vi "Client Example.vi"() -> ()   [LabVIEW 2016]
uses:
  <vilib>/NI/STM/SubVIs/MetaDataElement.ctl
  <vilib>/NI/STM/TCP/Read Meta Data (TCP Ref).vi
  <vilib>/NI/STM/TCP/Get Connection Reference (TCP).vi
  <vilib>/NI/STM/TCP/Read Meta Data (TCP Clst).vi
  <vilib>/NI/STM/TCP/Write Message (TCP).vi
  <vilib>/NI/STM/TCP/Read Message (TCP).vi
  <vilib>/NI/STM/NI STM.lvlib
panel:
  out "meta data":T1[](array[typedef])
  in  "Target IP Address":string="localhost"
  in  "Send":bool
  in  "Command":string
  in  "stop":bool
  out "command data string":string
  out "command name":string
  out "error  out":errorcluster
  # "ACTION"
  # "DEBUG"
  # "Set Server IP address (localhost default). \nRun VI. \nSend commands using SEND button, \nreceive ACKs in Debug indicators"
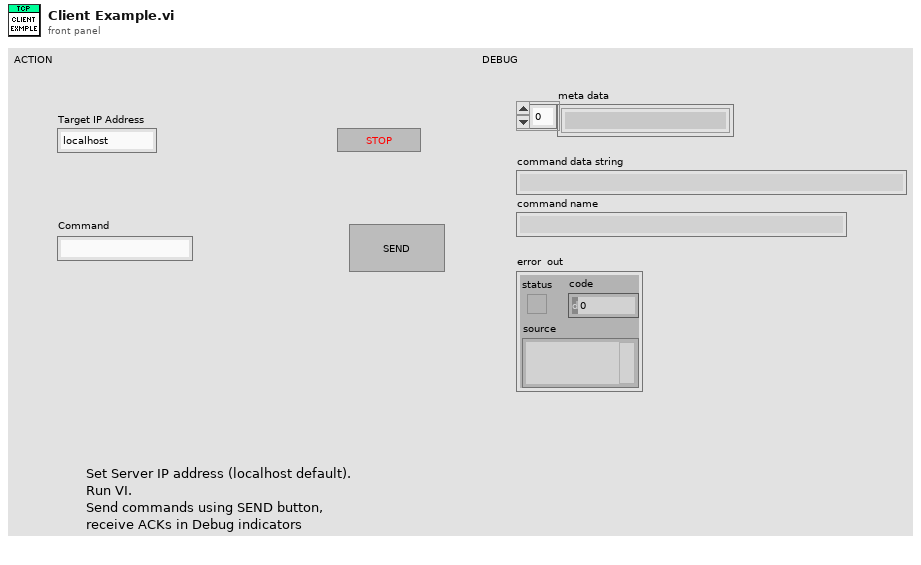
[diagram p1: front panel]
types:
  T1 = typedef "NI STM.lvlib/MetaDataElement.ctl" = string
  T2 = typedef "NI STM.lvlib/TCP Connection Info.ctl" = cluster{"connection ID":refnum<k5>, "meta data":T1[]}
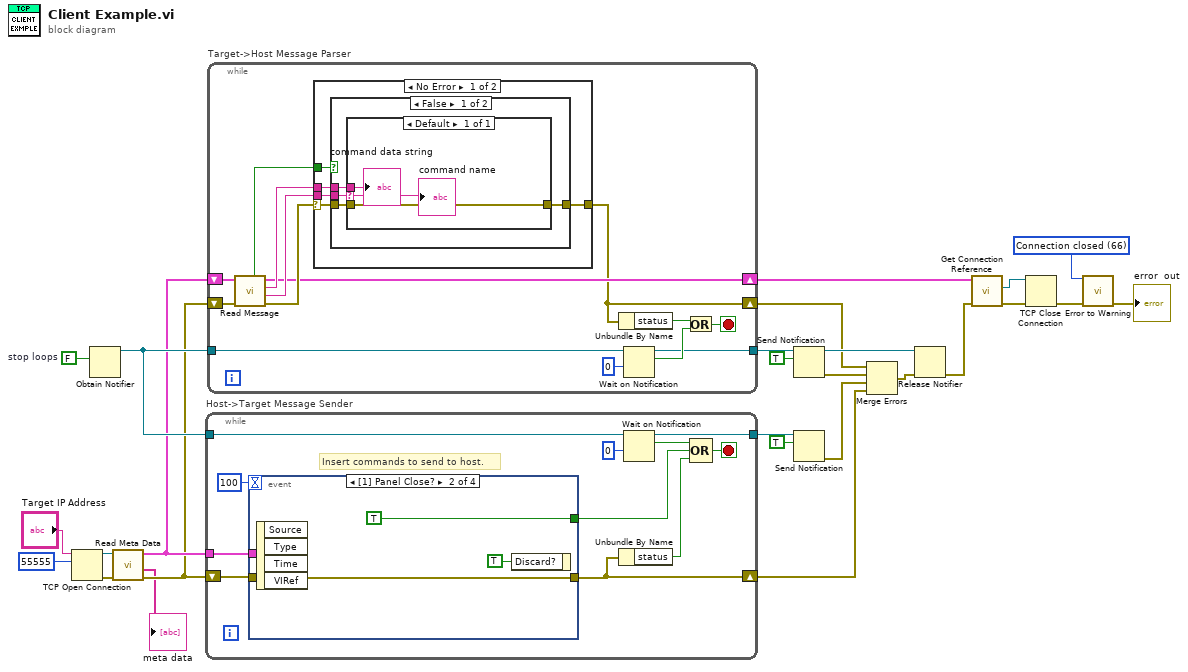
[diagram p0: block diagram]
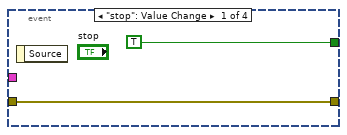
[diagram p2: hidden frame]
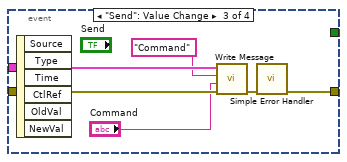
[diagram p3: hidden frame]
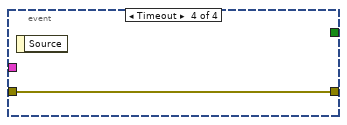
[diagram p4: hidden frame]
diagram:
  w12 = FALSE  # stop loops
  w24 = 66 items=["No Error", "Argument Error", "Memory Full", "Out of Zone", "End of File", "File Already Open", "Generic File IO Error", "File Not Found", "File Permission Error", "Disk Full", "Duplicate Path", "Too Many Files Open", "Not Enabled", "Resource File Not Found", "Cannot Add Resource", "Resource Not Found", "Image Not Found", "Image Memory Error", "Pen Does Not Exist", "Config Bad Type", "Config Token Not Found", "Config Parse Error", "Config Memory Error", "Bad External Code Format", "Bad External Code Offset", "External Code Not Present", "Null Window", "Destroy Window Mixup", "Null Menu", "Print Aborted", "Bad Print Record", "Print Driver Error", "Windows Error During Print", "Memory Error During Print", "Print Dialog Error", "Generic Print Error", "Invalid Device Refnum", "Device Not Found", "Device Parameter Error", "Device Unit Error", "Can't Open Device", "Device Call Aborted", "Generic Error", "Cancelled By User", "Object ID Too Low", "Object ID Too High", "Object Not In Heap", "Unknown Heap", "Bad DefProc ID", "DefProc Not In Table", "Message Out Of Range", "Null Method", "Unknown Message", "Manager Call Not Supported", "Bad address", "Connection In progress", "Connection timed out", "Connection is already in progress", "Network attribute not supported", "Network error", "Address in use", "System out of memory", "Connection aborted", "Connection refused", "Connection is not connected", "Connection is already connected", "Connection closed", "Initialize error (interapplication manager)", "Bad occurrence", "Wait on unbound occurrence handler", "Occurrence queue overflow", "Bad path", "Semaphore not signaled", "Unrecognized type (interapplication manager)"] ("1st Error to Convert")
  n1 = TCP Open Connection(address="Target IP Address", remote port or service name=u16 55555 ("remote port")) -> (connection ID=w8:refnum<k5>, error out=w7:errorcluster)  [unwired: 1 in, 2 out]
  n2 = Obtain Notifier(notification data type=w12) -> (notifier out=w15:refnum<notifier>)  [unwired: 3 in, 2 out]
  n3 = call-poly <vilib>:"Read Meta Data.vi"("error in"=w7, "connection ID"=w8) -> ("error out"=w9:errorcluster, "meta data"=→"meta data":T1[], "connection info out"=w10:T2)  [unwired: 1 in, 6 out]
  n4 = while "Host->Target Message Sender" {
    shift-right: [w29] -> w18
    shift-left: w9 -> [w37]
    tunnel: w10 -> [w36]
    tunnel: w15 -> [w33]
    tunnel: [w30] -> w16
    stop <- w31 stop-if-true
    # "Insert commands to send to host."
    n5 = event shown="[1] Panel Close?" {
      selector: _ -> [_ _ _ _]
      dyn-events: _ -> [_ _ _ _]
      timeout: 100 -> [_ _ _ _]
      tunnel: w36 -> [_ _ w48 _]
      tunnel: w37 -> [w39 w42 w47 w49]
      tunnel: [TRUE ("stop") TRUE ("stop") _ _] -> w28
      tunnel: [w39 w42 w45 w49] -> w29
      event "stop": Value Change {
        n6 = event-data() -> ()  [unwired: 2 out]
      }
      event Panel Close? {
        n7 = event-data() -> ()  [unwired: 5 out]
        n8 = event-data("Discard?"=TRUE) -> ()  [unwired: 1 in, 1 out]
      }
      event "Send": Value Change {
        n9 = event-data() -> ()  [unwired: 7 out]
        n10 = call-poly <vilib>:"Write Message.vi"("error in"=w47, "data"="Command", "name"="Command", "connection info in"=w48) -> ("error out"=w46:errorcluster)  [unwired: 1 in, 6 out]
        n11 = call <vilib>:"Simple Error Handler.vi"("error in (no error)"=w46) -> ("error out"=w45:errorcluster)  [unwired: 4 in, 4 out]
      }
      event Timeout {
        n12 = event-data() -> ()  [unwired: 2 out]
      }
    }
    n13 = Unbundle By Name(w29) -> ("status"=w27:bool)
    n14 = Wait on Notification(notifier=w33, timeout in ms (-1)=0) -> (notifier out=w30:refnum<notifier>, notification=w35:bool)  [unwired: 2 in, 2 out]
    n15 = Compound Arithmetic op=OR(w35, w28, w27) -> (w31:bool)
  }
  n16 = while "Target->Host Message Parser" {
    shift-right: [w50] -> w4
    shift-left: w9 -> [w62]
    tunnel: w15 -> [w56]
    tunnel: [w52] -> w13
    shift-right: [w57] -> w11
    shift-left: w10 -> [w63]
    stop <- w53 stop-if-true
    n17 = call-poly <vilib>:"Read Message.vi"("error in"=w62, "connection info in"=w63) -> ("error out"=w58:errorcluster, "name"=w61:T1, "data string"=w60:string, "connection info out"=w57:T2, "timed out?"=w59:bool)  [unwired: 3 in, 2 out]
    n18 = case shown="No Error" w58 {
      selector: w58 -> [w65 w77]
      tunnel: w61 -> [w68 _]
      tunnel: w60 -> [w67 _]
      tunnel: w59 -> [w66 _]
      tunnel: [w64 w77] -> w50
      frame No Error {
        n19 = case shown="False" w66 {
          tunnel: w68 -> [w69 _]
          tunnel: w67 -> [w72 _]
          tunnel: w65 -> [w71 w76]
          tunnel: [w70 w76] -> w64
          frame False {
            n20 = case shown="Default" w69 {
              selector: w69 -> [w73]
              tunnel: w72 -> [w74]
              tunnel: w71 -> [w75]
              tunnel: [w75] -> w70
              frame Default {
                "command data string" <- w74
                "command name" <- w73
              }
            }
          }
          frame True {
          }
        }
      }
      frame Error {
      }
    }
    n21 = Unbundle By Name(w50) -> ("status"=w51:bool)
    n22 = Wait on Notification(notifier=w56, timeout in ms (-1)=0) -> (notifier out=w52:refnum<notifier>, notification=w54:bool)  [unwired: 2 in, 2 out]
    n23 = Or(x=w51, y=w54) -> (x .or. y?=w53:bool)
  }
  n24 = Send Notification(notification=TRUE, notifier=w13) -> (notifier out=w21:refnum<notifier>, error out=w20:errorcluster)  [unwired: 1 in]
  n25 = Send Notification(notification=TRUE, notifier=w16) -> (error out=w19:errorcluster)  [unwired: 1 in, 1 out]
  n26 = Merge Errors(w4, w20, w19, w18) -> (w22:errorcluster)
  n27 = Release Notifier(notifier=w21, error in (no error)=w22) -> (error out=w23:errorcluster)  [unwired: 1 in, 2 out]
  n28 = call-poly <vilib>:"Get Connection Reference.vi"("error in"=w23, "connection info in"=w11) -> ("error out"=w3:errorcluster, "connection ID out"=w2:refnum<k5>)  [unwired: 8 out]
  n29 = TCP Close Connection(connection ID=w2, error in (no error)=w3) -> (error out=w25:errorcluster)  [unwired: 2 out]
  n30 = call <vilib>:"Error to Warning.vi"("1st Error to Convert"=w24, "error in"=w25) -> ("warning out"=→"error  out":errorcluster)  [unwired: 3 in, 10 out]
